vi "UI-InitialParam.vi"(5 "名称或相对路径":string, 11 "error in (no error)":errorcluster caption="错误输入（无错误）") -> (4 "ParamsUI 侧面 Out":T11 {"Rectangle"."Rotation" format="%.2f"; "Rectangle"."Left" scale=0.0..1024.0; "Rectangle"."Right" scale=0.0..1024.0}, 6 "ParamsUI 正面":T9, 8 "图片处理效果参数 正面":T8={"二值化参数"={"Lower value"=169.0, "Upper value"=255.0}, "形态学分析模式"=enum."Erode", "形态学 迭代次数"=3, "特殊分析-滤波"=[{"Measurement Parameter"=19, "Range Lower Value"=0.0, "Range Upper Value"=1300.0, "Range"=FALSE, "Measurement Type"=FALSE}], "特殊分析-移除/保留"=TRUE} {"特殊分析-滤波"."Measurement Parameter" items=["Center of Mass X", "Center of Mass Y", "First Pixel X", "First Pixel Y", "Bounding Rect Left", "Bounding Rect Top", "Bounding Rect Right", "Bounding Rect Bottom", "Max Feret Diameter Start X", "Max Feret Diameter Start Y", "Max Feret Diameter End X", "Max Feret Diameter End Y", "Max Horiz. Segment Length Left", "Max Horiz. Segment Length Right", "Max Horiz. Segment Length Row", "-", "Bounding Rect Width", "Bounding Rect Height", "Bounding Rect Diagonal", "Perimeter", "Convex Hull Perimeter", "Holes' Perimeter", "Max Feret Diameter", "Equivalent Ellipse Major Axis", "Equivalent Ellipse Minor Axis", "Equivalent Ellipse Minor Axis (Feret)", "Equivalent Rect Long Side", "Equivalent Rect Short Side", "Equivalent Rect Diagonal", "Equivalent Rect Short Side (Feret)", "Average Horiz. Segment Length", "Average Vert. Segment Length", "Hydraulic Radius", "Waddel Disk Diameter", "-", "Area", "Holes' Area", "Particle & Holes' Area", "Convex Hull Area", "Image Area", "-", "Number of Holes", "Number of Horiz. Segments", "Number of Vert. Segments", "-", "Orientation", "Max Feret Diameter Orientation", "-", "% Area/Image Area", "% Area/(Particle & Holes' Area)", "Ratio of Equivalent Ellipse Axes", "Ratio of Equivalent Rect Sides", "-", "Elongation Factor", "Compactness Factor", "Heywood Circularity Factor", "Type Factor", "-", "Sum X", "Sum Y", "Sum XX", "Sum XY", "Sum YY", "Sum XXX", "Sum XXY", "Sum XYY", "Sum YYY", "-", "Moment of Inertia XX", "Moment of Inertia XY", "Moment of Inertia YY", "Moment of Inertia XXX", "Moment of Inertia XXY", "Moment of Inertia XYY", "Moment of Inertia YYY", "Norm. Moment of Inertia XX", "Norm. Moment of Inertia XY", "Norm. Moment of Inertia YY", "Norm. Moment of Inertia XXX", "Norm. Moment of Inertia XXY", "Norm. Moment of Inertia XYY", "Norm. Moment of Inertia YYY", "Hu Moment 1", "Hu Moment 2", "Hu Moment 3", "Hu Moment 4", "Hu Moment 5", "Hu Moment 6", "Hu Moment 7"]}, 10 "定位分析参数设定 正面":T7={"是否启动图片分析"=FALSE, "定位圆环ROI"={"Center X"=0, "Center Y"=0, "Inner Radius"=0, "Outer Radius"=0, "Start Angle"=0.0, "End Angle"=0.0}, "圆环Options "={"Process"=enum."Get First Edge", "Step Size"=20, "Max Pixel Radius"=3}, "Options (Find Circular)"={"Search  Direction"=1, "Edge Options"={"Edge Polarity"=0, "Kernel Size"=3, "Width"=3, "Minimum Edge Strength"=178.0, "Interpolation Type"=enum."Bilinear Fixed", "Data Processing Method"=enum."Average"}, "Show Search Area"=TRUE, "Show Search Lines"=TRUE, "Show Edges Found"=TRUE, "Show Result"=TRUE, "Search Area Color"=65280, "Search Lines Color"=255, "Edge Locations Color"=16776960, "Result Color"=16711680, "Overlay Group Name"=""}} {"Options (Find Circular)"."Search  Direction" items=["Outside to Inside", "Inside to Outside"]; "Options (Find Circular)"."Edge Options"."Edge Polarity" items=["All Edges", "Rising Edges", "Falling Edges"]; "Options (Find Circular)"."Edge Options"."Minimum Edge Strength" format="%.2f"; "Options (Find Circular)"."Edge Options"."Width" step=2; "Options (Find Circular)"."Edge Options"."Kernel Size" step=2; "定位圆环ROI"."End Angle" min=-90.0 max=90.0 step=1.0 format="%.2f"; "定位圆环ROI"."Start Angle" min=-90.0 max=90.0 step=1.0 format="%.2f"; "定位圆环ROI"."Center X" scale=0.0..1024.0}, 14 "分析参数设定 正面":T4={"溢出距离下限"="", "溢出距离上限"="", "像素分辨率"="", "Search Direction "=enum."Annulus Outer To Inner", "Curve Extraction "={"Extraction Mode"=0, "Edge Threshold"=75, "Edge Filter Size"=0, "Min Length"=25, "Search Step Size"=15, "Max Endpoint Gap"=10, "Subpixel"=TRUE}, "Contour Selection "=enum."Closest To Search Start", "Curve Connection "=[{"Match Constraints"=0, "Min"=1.0, "Max"=12.0}], "Kernel Width "=5, "Curve Extraction 2 "={"Extraction Mode"=0, "Edge Threshold"=75, "Edge Filter Size"=0, "Min Length"=25, "Search Step Size"=15, "Max Endpoint Gap"=10, "Subpixel"=TRUE}, "Match Mode "={"Rotation"=FALSE, "Scale"=FALSE, "Occlusion"=FALSE}, "Smoothing Kernel "=0, "Template File Path "=path "C:/Users/hedongpo/Desktop/吕亚/Temp3.png", "Circle or Annulus"={"Center X"=0, "Center Y"=0, "Inner Radius"=0, "Outer Radius"=0, "Start Angle"=0.0, "End Angle"=0.0}} {"Circle or Annulus"."End Angle" min=-90.0 max=90.0 step=1.0 format="%.2f"; "Circle or Annulus"."Start Angle" min=-90.0 max=90.0 step=1.0 format="%.2f"; "Circle or Annulus"."Center X" scale=0.0..1024.0; "Curve Extraction"."Extraction Mode" items=["Normal", "Uniform Regions"]; "Curve Extraction"."Edge Filter Size" items=["Fine", "Normal", "Contour Tracing"]; "Curve Extraction"."Max Endpoint Gap" min=0; "Curve Extraction"."Search Step Size" min=1 max=255 step=1; "Curve Extraction"."Min Length" min=0; "Curve Extraction"."Edge Threshold" min=1 max=350 step=1; "Curve Connection"."Max" format="%.2f"; "Curve Connection"."Min" format="%.2f"; "Curve Connection"."Match Constraints" items=["Distance (pixel)", "Angle Difference (degrees)", "Connectivity Distance (pixel)", "Gradient Difference (degrees)"]; "Curve Extraction 2"."Extraction Mode" items=["Normal", "Uniform Regions"]; "Curve Extraction 2"."Edge Filter Size" items=["Fine", "Normal", "Contour Tracing"]; "Curve Extraction 2"."Max Endpoint Gap" min=0; "Curve Extraction 2"."Search Step Size" min=1 max=255 step=1; "Curve Extraction 2"."Min Length" min=0; "Curve Extraction 2"."Edge Threshold" min=1 max=350 step=1}, 15 "错误输出":errorcluster)   [LabVIEW 2017]
uses:
  <vilib>/vision/Measure.llb/Edge Options.ctl
  <vilib>/vision/Measure.llb/Edge Polarity.ctl
  <vilib>/vision/Contour.llb/IMAQ Contour Curve Extraction.ctl
  <vilib>/vision/Contour.llb/IMAQ Connect Range Setting.ctl
  Global System.vi
  <vilib>/Utility/xml.llb/Read From XML File(string).vi
panel:
  out "添加的路径":path
  # "D:\\KNight Back Housing\\Source Code\\Template Program\\potteryTemplete"
  # "Range"
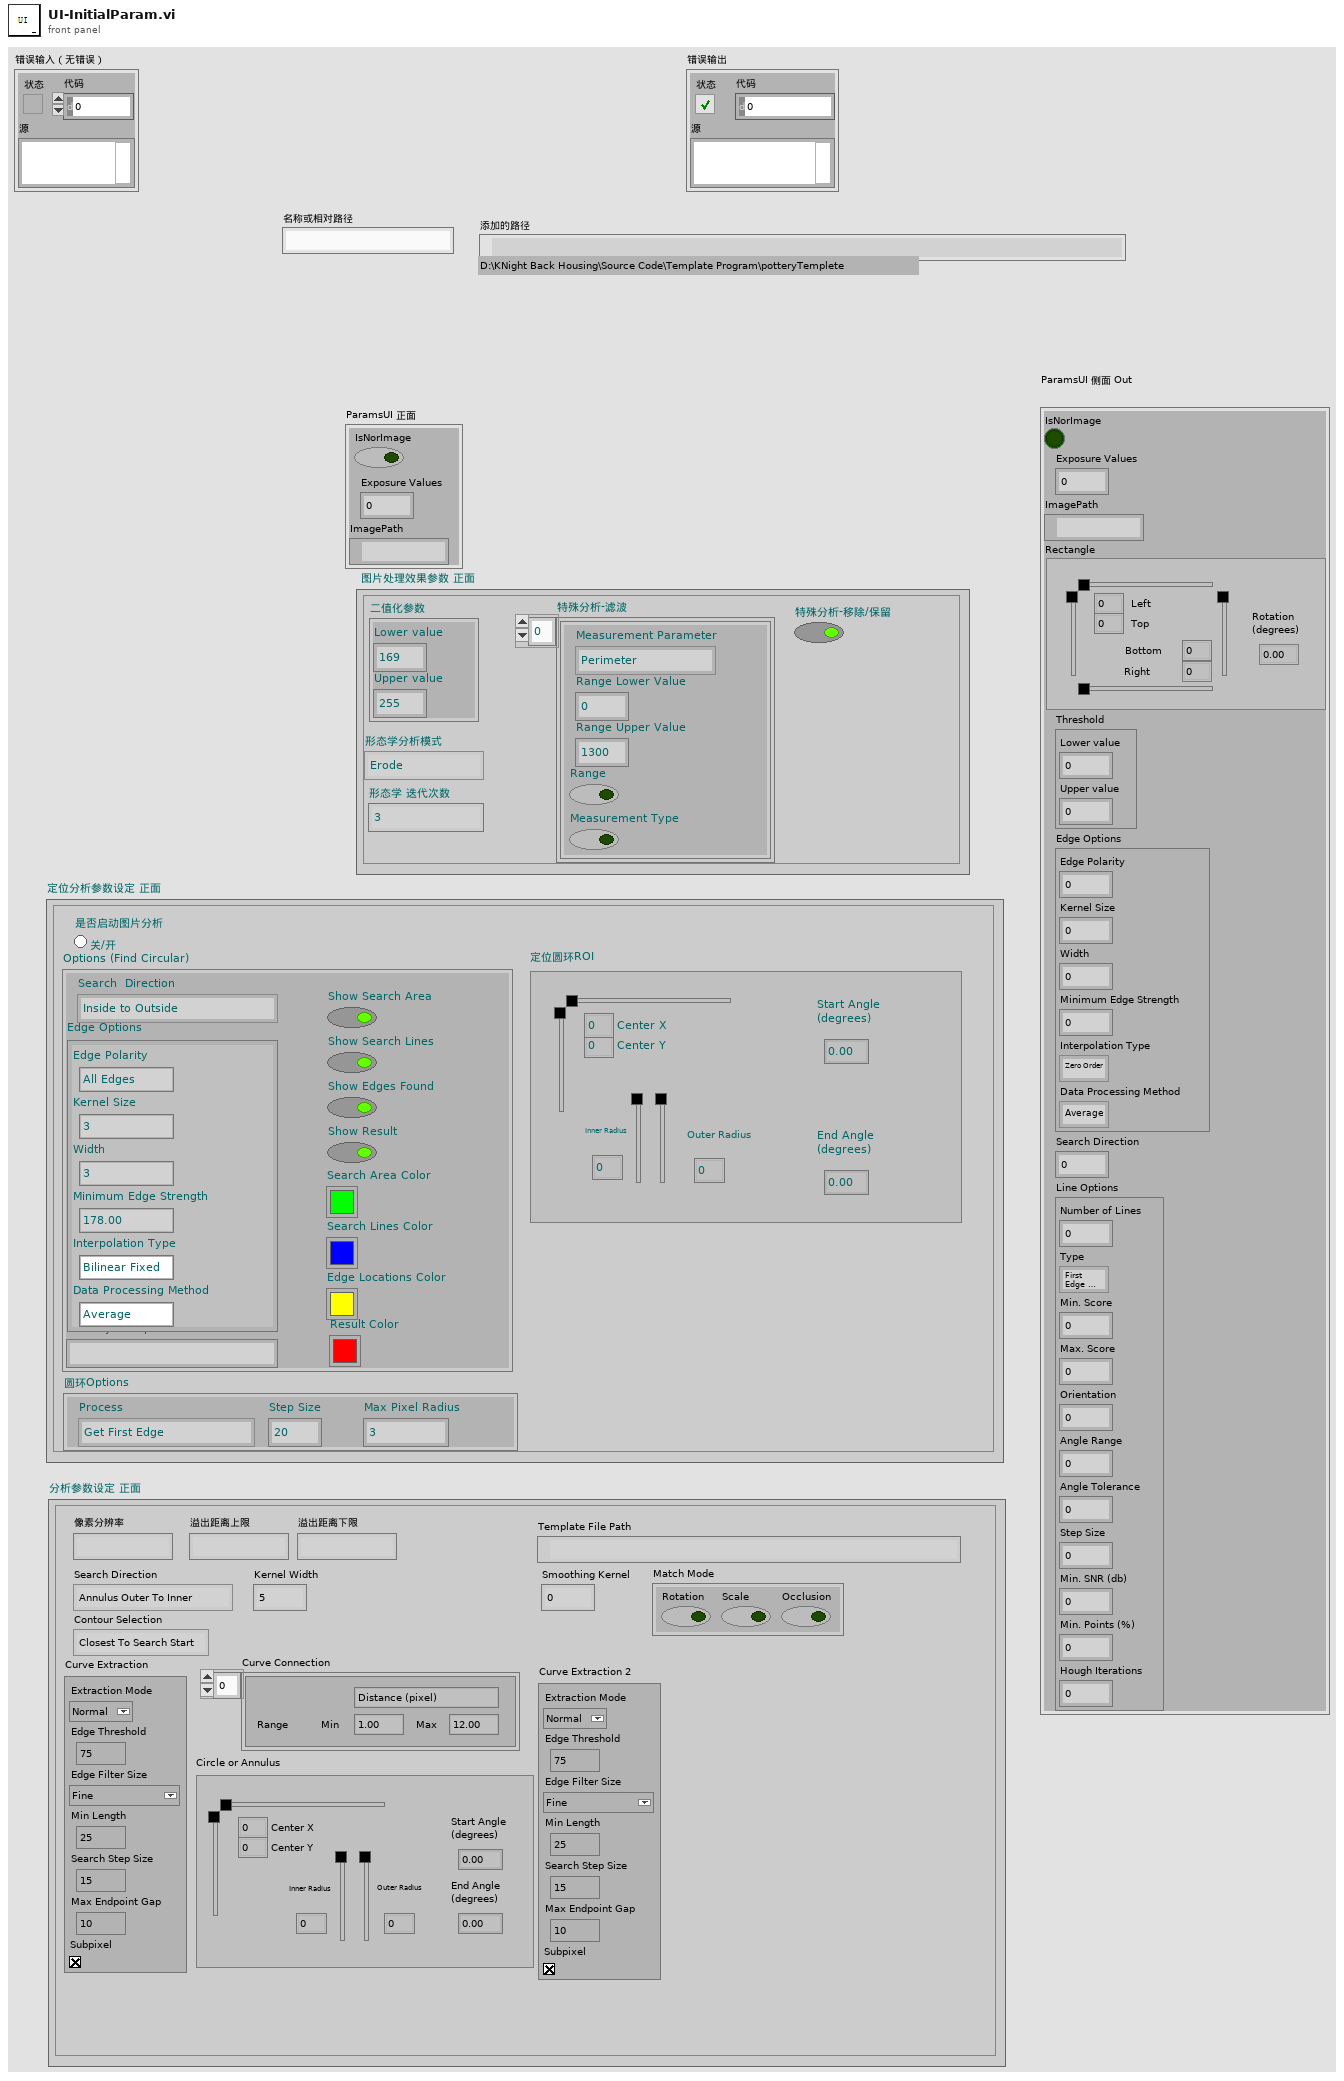
[diagram p1: front panel]
types:
  T1 = typedef "IMAQ Contour Curve Extraction.ctl" = cluster{"Extraction Mode":u32, "Edge Threshold":i32, "Edge Filter Size":u32, "Min Length":i32, "Search Step Size":i32, "Max Endpoint Gap":i32, "Subpixel":bool}
  T2 = typedef "IMAQ Connect Range Setting.ctl" = cluster{"Match Constraints":u32, "Min":dbl, "Max":dbl}
  T3 = typedef "IMAQ Circle" = cluster{"Center X":i32, "Center Y":i32, "Inner Radius":i32, "Outer Radius":i32, "Start Angle":dbl, "End Angle":dbl}
  T4 = cluster{"溢出距离下限":string, "溢出距离上限":string, "像素分辨率":string, "Search Direction ":enum16{"Rect Left To Right", "Rect Right To Left", "Rect Top To Bottom", "Rect Bottom To Top", "Annulus Inner To Outer", "Annulus Outer To Inner", "Annulus Start Angle To End Angle", "Annulus End Angle To Start Angle"}, "Curve Extraction ":T1, "Contour Selection ":enum16{"Closest To Search Start", "Maximum Length", "Strongest Mean Gradient Change"}, "Curve Connection ":T2[], "Kernel Width ":u32, "Curve Extraction 2 ":T1, "Match Mode ":cluster{"Rotation":bool, "Scale":bool, "Occlusion":bool}, "Smoothing Kernel ":u32, "Template File Path ":path, "Circle or Annulus":T3}
  T5 = typedef "Edge Options.ctl" = cluster{"Edge Polarity":T6, "Kernel Size":u32, "Width":u32, "Minimum Edge Strength":sgl, "Interpolation Type":enum32{"Zero Order", "Bilinear", "Quadratic", "Cubic", "Bilinear Fixed"}, "Data Processing Method":enum32{"Average", "Median"}}
  T6 = typedef "Edge Polarity.ctl" = u32
  T7 = cluster{"是否启动图片分析":bool, "定位圆环ROI":T3, "圆环Options ":cluster{"Process":enum16{"Get First Edge", "Get First + Last Edge", "Get All Edges", "Get Best Edge"}, "Step Size":i32, "Max Pixel Radius":i32}, "Options (Find Circular)":cluster{"Search  Direction":u32, "Edge Options":T5, "Show Search Area":bool, "Show Search Lines":bool, "Show Edges Found":bool, "Show Result":bool, "Search Area Color":u32, "Search Lines Color":u32, "Edge Locations Color":u32, "Result Color":u32, "Overlay Group Name":string}}
  T8 = cluster{"二值化参数":cluster{"Lower value":sgl, "Upper value":sgl}, "形态学分析模式":enum32{"AutoM", "Close", "Dilate", "Erode", "Gradient", "Gradient out", "Gradient in", "Hit miss", "Open", "PClose", "POpen", "Thick", "Thin"}, "形态学 迭代次数":i32, "特殊分析-滤波":cluster{"Measurement Parameter":i32, "Range Lower Value":dbl, "Range Upper Value":dbl, "Range":bool, "Measurement Type":bool}[], "特殊分析-移除/保留":bool}
  T9 = cluster{"IsNorImage":bool, "Exposure Values":u32, "ImagePath":path}
  T10 = typedef "IMAQ Rectangle" = cluster{"Left":i32, "Top":i32, "Right":i32, "Bottom":i32, "Rotation":dbl}
  T11 = cluster{"IsNorImage":bool, "Exposure Values":u32, "ImagePath":path, "Rectangle":T10, "Threshold ":cluster{"Lower value":sgl, "Upper value":sgl}, "Edge Options ":cluster{"Edge Polarity":u32, "Kernel Size":u32, "Width":u32, "Minimum Edge Strength":sgl, "Interpolation Type":enum32{"Zero Order", "Bilinear", "Quadratic", "Cubic", "Bilinear Fixed"}, "Data Processing Method":enum32{"Average", "Median"}}, "Search Direction":u32, "Line Options":cluster{"Number of Lines":i32, "Type":enum32{"First Edge Rake", "Best Edge Rake", "Hough Edge Rake", "First Edge Projection", "Best Edge Projection"}, "Min. Score":dbl, "Max. Score":dbl, "Orientation":dbl, "Angle Range":dbl, "Angle Tolerance":dbl, "Step Size":u32, "Min. SNR (db)":dbl, "Min. Points (%)":dbl, "Hough Iterations":i32}}
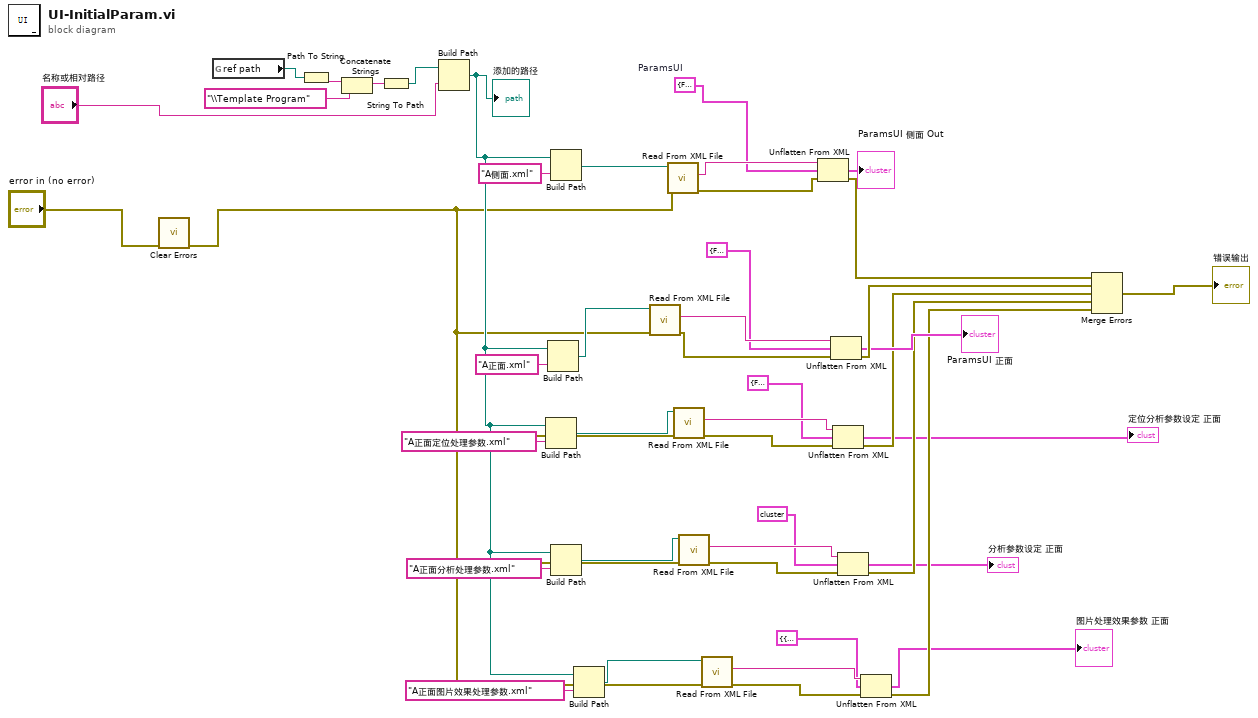
[diagram p0: block diagram]
diagram:
  w36 = T11 {"IsNorImage"=FALSE, "Exposure Values"=0, "ImagePath"=path "", "Rectangle"={"Left"=0, "Top"=0, "Right"=0, "Bottom"=0, "Rotation"=0.0}, "Threshold "={"Lower value"=130.0, "Upper value"=255.0}, "Edge Options "={"Edge Polarity"=1, "Kernel Size"=13, "Width"=9, "Minimum Edge Strength"=104.32, "Interpolation Type"=enum."Zero Order", "Data Processing Method"=enum."Average"}, "Search Direction"=2, "Line Options"={"Number of Lines"=10, "Type"=enum."Hough Edge Rake", "Min. Score"=0.0, "Max. Score"=1024.0, "Orientation"=0.0, "Angle Range"=20.0, "Angle Tolerance"=1.0, "Step Size"=19, "Min. SNR (db)"=15.0, "Min. Points (%)"=25.0, "Hough Iterations"=20}}  # ParamsUI
  n1 = call <vilib>:"Clear Errors.vi"("error in (no error)"="error in (no error)") -> ("error out"=w7:errorcluster)  [unwired: 5 in, 1 out]
  n2 = global read "Global System.vi" "ref path"() -> (w42:path)
  n3 = Path To String(path=w42) -> (string=w45:string)
  n4 = Concatenate Strings(w45, "\\Template Program" ("字符串")) -> (w43:string)
  n5 = String To Path(string=w43) -> (path=w41:path)
  n6 = Build Path(base path=w41, name or relative path="名称或相对路径") -> (appended path=w10:path)
  "添加的路径" <- w10
  n7 = Build Path(base path=w10, name or relative path="A正面定位处理参数.xml" ("名称或相对路径")) -> (appended path=w23:path)
  n8 = Build Path(base path=w10, name or relative path="A正面.xml" ("名称或相对路径")) -> (appended path=w30:path)
  n9 = Build Path(base path=w10, name or relative path="A侧面.xml" ("名称或相对路径")) -> (appended path=w38:path)
  n10 = Build Path(base path=w10, name or relative path="A正面分析处理参数.xml" ("名称或相对路径")) -> (appended path=w17:path)
  n11 = Build Path(base path=w10, name or relative path="A正面图片效果处理参数.xml" ("名称或相对路径")) -> (appended path=w9:path)
  n12 = call-poly <vilib>:"Read From XML File.vi"("error in (no error)"=w7, "XML File Path"=w30) -> ("error out"=w27:errorcluster, "XML Elements"=w29:string)  [unwired: 7 in, 1 out]
  n13 = call-poly <vilib>:"Read From XML File.vi"("error in (no error)"=w7, "XML File Path"=w38) -> ("error out"=w35:errorcluster, "XML Elements"=w37:string)  [unwired: 7 in, 1 out]
  n14 = call-poly <vilib>:"Read From XML File.vi"("error in (no error)"=w7, "XML File Path"=w23) -> ("error out"=w21:errorcluster, "XML Elements"=w22:string)  [unwired: 7 in, 1 out]
  n15 = call-poly <vilib>:"Read From XML File.vi"("error in (no error)"=w7, "XML File Path"=w17) -> ("error out"=w19:errorcluster, "XML Elements"=w18:string)  [unwired: 7 in, 1 out]
  n16 = call-poly <vilib>:"Read From XML File.vi"("error in (no error)"=w7, "XML File Path"=w9) -> ("error out"=w12:errorcluster, "XML Elements"=w13:string)  [unwired: 7 in, 1 out]
  n17 = Unflatten From XML(xml string=w37, type=w36, error in (no error)=w35) -> (value=→"ParamsUI 侧面 Out":T11, error out=w33:errorcluster)
  n18 = Unflatten From XML(xml string=w29, type=T9 {"IsNorImage"=FALSE, "Exposure Values"=0, "ImagePath"=path ""} ("ParamsUI 正面"), error in (no error)=w27) -> (value=→"ParamsUI 正面":T9, error out=w26:errorcluster)
  n19 = Unflatten From XML(xml string=w22, type=T7 {"是否启动图片分析"=FALSE, "定位圆环ROI"={"Center X"=0, "Center Y"=0, "Inner Radius"=0, "Outer Radius"=0, "Start Angle"=0.0, "End Angle"=0.0}, "圆环Options "={"Process"=enum."Get First Edge", "Step Size"=20, "Max Pixel Radius"=3}, "Options (Find Circular)"={"Search  Direction"=1, "Edge Options"={"Edge Polarity"=0, "Kernel Size"=3, "Width"=3, "Minimum Edge Strength"=178.0, "Interpolation Type"=enum."Bilinear Fixed", "Data Processing Method"=enum."Average"}, "Show Search Area"=TRUE, "Show Search Lines"=TRUE, "Show Edges Found"=TRUE, "Show Result"=TRUE, "Search Area Color"=65280, "Search Lines Color"=255, "Edge Locations Color"=16776960, "Result Color"=16711680, "Overlay Group Name"=""}} ("定位分析参数设定 正面"), error in (no error)=w21) -> (value=→"定位分析参数设定 正面":T7, error out=w20:errorcluster)
  n20 = Unflatten From XML(xml string=w18, type=T4 {"溢出距离下限"="", "溢出距离上限"="", "像素分辨率"="", "Search Direction "=enum."Annulus Outer To Inner", "Curve Extraction "={"Extraction Mode"=0, "Edge Threshold"=75, "Edge Filter Size"=0, "Min Length"=25, "Search Step Size"=15, "Max Endpoint Gap"=10, "Subpixel"=TRUE}, "Contour Selection "=enum."Closest To Search Start", "Curve Connection "=[{"Match Constraints"=0, "Min"=1.0, "Max"=12.0}], "Kernel Width "=5, "Curve Extraction 2 "={"Extraction Mode"=0, "Edge Threshold"=75, "Edge Filter Size"=0, "Min Length"=25, "Search Step Size"=15, "Max Endpoint Gap"=10, "Subpixel"=TRUE}, "Match Mode "={"Rotation"=FALSE, "Scale"=FALSE, "Occlusion"=FALSE}, "Smoothing Kernel "=0, "Template File Path "=path "C:/Users/hedongpo/Desktop/吕亚/Temp3.png", "Circle or Annulus"={"Center X"=0, "Center Y"=0, "Inner Radius"=0, "Outer Radius"=0, "Start Angle"=0.0, "End Angle"=0.0}} ("分析参数设定 正面"), error in (no error)=w19) -> (value=→"分析参数设定 正面":T4, error out=w15:errorcluster)
  n21 = Unflatten From XML(xml string=w13, type=T8 {"二值化参数"={"Lower value"=169.0, "Upper value"=255.0}, "形态学分析模式"=enum."Erode", "形态学 迭代次数"=3, "特殊分析-滤波"=[{"Measurement Parameter"=19, "Range Lower Value"=0.0, "Range Upper Value"=1300.0, "Range"=FALSE, "Measurement Type"=FALSE}], "特殊分析-移除/保留"=TRUE} ("图片处理效果参数 正面"), error in (no error)=w12) -> (value=→"图片处理效果参数 正面":T8, error out=w11:errorcluster)
  n22 = Merge Errors(w33, w26, w20, w15, w11) -> (→"错误输出":errorcluster)
